vi "Factorial Sub Vi.vi"(11 "Numeric in":i32) -> (3 "Numeric out":i32)   [LabVIEW 2020]
doc: "This is Factorial VI you need to enter anu numeric then got Factorial result"
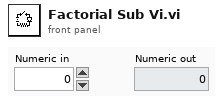
[diagram p1: front panel]
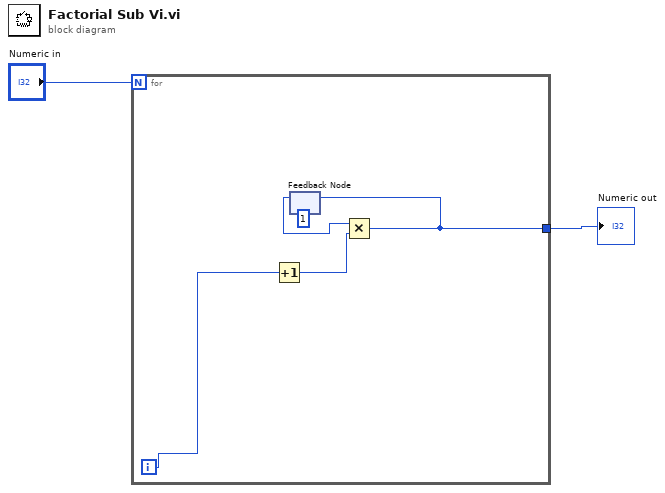
[diagram p0: block diagram]
diagram:
  n1 = for {
    N: "Numeric in" -> [_]
    tunnel: [w3] -> w1
    i -> [w6]
    n2 = Increment(x=w6) -> (x+1=w7:i32)
    n3 = feedback #1(1) -> (w5:i32)
    n4 = Multiply(x=w5, y=w7) -> (x*y=w3:i32)
    n5 = feedback-in #1(w3) -> ()
  }
  "Numeric out" <- w1
